vi "ApplyFilter.vi"(9 "Filter":cluster{"Matches String":string, "Column":i32}[](array[cluster]), 10 "Mode":enum8{"AND", "OR", "NOT AND", "NOT OR"}(ring), 11 "Tree":T1[](array[typedef])) -> (3 "Array":T1[](array[typedef]))   [LabVIEW 2021, in "Tree.lvlib" / "Tree.lvclass"]
uses:
  Tree.lvclass
  TreeData.ctl
  Tree.lvclass/Tree.ctl
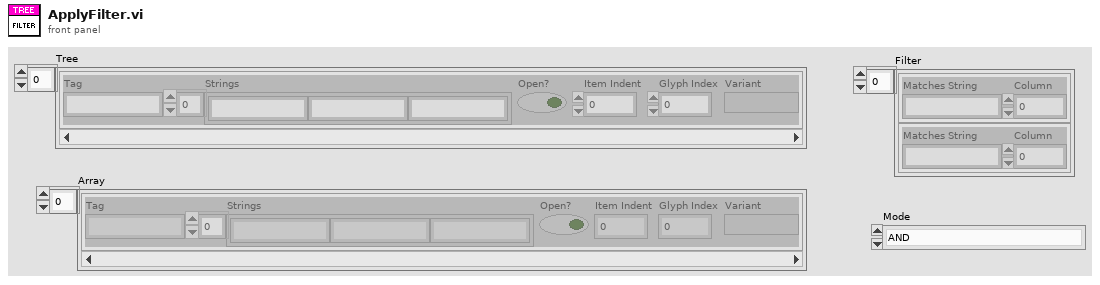
[diagram p1: front panel]
types:
  T1 = typedef "Tree.lvlib/Tree.lvclass/TreeData.ctl" = cluster{"Tag":string, "Strings":string[], "Open?":bool, "Item Indent":i32, "Glyph Index":i32, "Variant":variant}
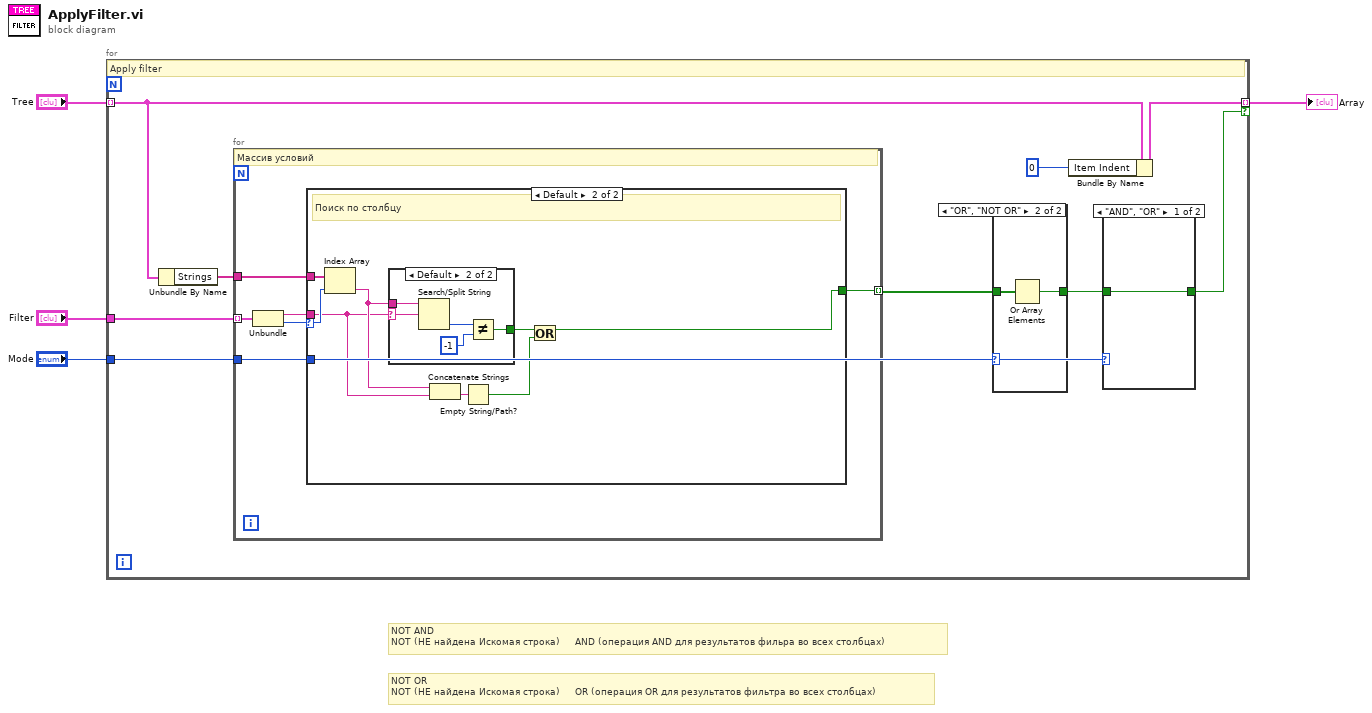
[diagram p0: block diagram]
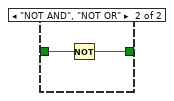
[diagram p2: hidden frame]
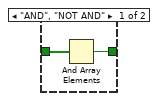
[diagram p3: hidden frame]
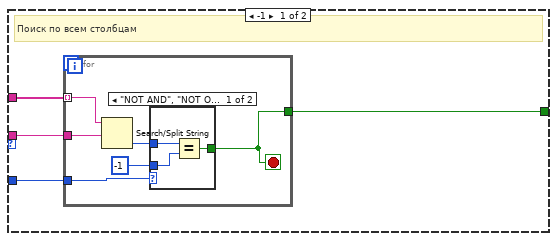
[diagram p4: hidden frame]
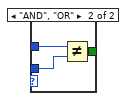
[diagram p5: hidden frame]
diagram:
  # "NOT OR\nNOT (НЕ найдена Искомая строка)     OR (операция OR для результатов фильтра во всех столбцах)"
  # "NOT AND\nNOT (НЕ найдена Искомая строка)     AND (операция AND для результатов фильра во всех столбцах)"
  n1 = for {
    tunnel: "Tree" -> [w11] mode=indexing
    tunnel: "Filter" -> [w13]
    tunnel: [w10] -> w2 mode=indexing if=w5
    tunnel: "Mode" -> [w7]
    # "Apply filter"
    n2 = Unbundle By Name(w11) -> ("Strings"=w12:string[])
    n3 = for {
      tunnel: w13 -> [w26] mode=indexing
      tunnel: w12 -> [w21]
      tunnel: [w23] -> w8 mode=indexing
      tunnel: w7 -> [w22]
      # "Массив условий"
      n4 = Unbundle(w26) -> ("Matches String"=w25:string, "Column"=w24:i32)
      n5 = case shown="Default" w24 {
        selector: w24 -> [_ w49]
        tunnel: w21 -> [w30 w50]
        tunnel: w25 -> [w29 w43]
        tunnel: [w28 w45] -> w23
        tunnel: w22 -> [w27 _]
        frame -1 {
          # "Поиск по всем столбцам"
          n6 = for {
            tunnel: w30 -> [w34] mode=indexing
            tunnel: w29 -> [w33]
            tunnel: [w32] -> w28
            tunnel: w27 -> [w31]
            stop <- w32 stop-if-true
            n7 = Search/Split String(string=w34, search string/char (-)=w33) -> (offset of match=w35:i32)  [unwired: 1 in, 2 out]
            n8 = case shown="\"NOT AND\", \"NOT OR\"" w31 {
              tunnel: -1 ("y") -> [w38 w42]
              tunnel: w35 -> [w39 w41]
              tunnel: [w37 w40] -> w32
              frame "NOT AND", "NOT OR" {
                n9 = Equal?(x=w39, y=w38) -> (x = y?=w37:bool)
              }
              frame "AND", "OR" {
                n10 = Not Equal?(x=w41, y=w42) -> (x != y?=w40:bool)
              }
            }
          }
        }
        frame Default {
          # "Поиск по столбцу"
          n11 = Index Array(array=w50, index=w49) -> (element=w48:string)
          n12 = case shown="Default" w43 {
            selector: w43 -> [_ w51]
            tunnel: w48 -> [_ w53]
            tunnel: [_ w52] -> w46
            frame "" {
            }
            frame Default {
              n13 = Search/Split String(string=w53, search string/char (-)=w51) -> (offset of match=w54:i32)  [unwired: 1 in, 2 out]
              n14 = Not Equal?(x=w54, y=-1) -> (x != y?=w52:bool)
            }
          }
          n15 = Concatenate Strings(w48, w43) -> (w47:string)
          n16 = Empty String/Path?(string/path=w47) -> (empty?=w44:bool)
          n17 = Or(x=w46, y=w44) -> (x .or. y?=w45:bool)
        }
      }
    }
    n18 = case shown="\"OR\", \"NOT OR\"" w7 {
      tunnel: w8 -> [w18 w20]
      tunnel: [w17 w19] -> w6
      frame "AND", "NOT AND" {
        n19 = And Array Elements(Boolean array=w18) -> (logical AND=w17:bool)
      }
      frame "OR", "NOT OR" {
        n20 = Or Array Elements(Boolean array=w20) -> (logical OR=w19:bool)
      }
    }
    n21 = Bundle By Name(cluster=w11, "Item Indent"=0) -> (w10:T1)
    n22 = case shown="\"AND\", \"OR\"" w7 {
      tunnel: [w14 w15] -> w5
      tunnel: w6 -> [w14 w16]
      frame "AND", "OR" {
      }
      frame "NOT AND", "NOT OR" {
        n23 = Not(x=w16) -> (.not. x?=w15:bool)
      }
    }
  }
  "Array" <- w2
